vi "GA_Apply Elitism.vi"(6 "Parameters":T2={"Population size"=100, "Generations no."=500, "Significant digits"=4, "Crossover probabality"=0.85, "Mutation mode"=enum."one-point, fixed rate", "Use Gray code?"=FALSE, "Mutation rate"=0.05, "Min mutation rate"=0.0005, "Max mutation rate"=0.25, "Reproduction plan"=enum."Steady-state-replace-worst", "Elitism"=FALSE, "Fmax"=1} {"Max mutation rate" min=0.0 max=1.0; "Min mutation rate" min=0.0 max=1.0; "Mutation rate" min=0.0 max=1.0; "Crossover probabality" min=0.0 max=1.0; "Significant digits" min=1; "Generations no." min=1; "Population size" min=1}, 10 "Old Population":T1, 11 "Population in":T1) -> (3 "Population out":T1)   [LabVIEW 2016, in "Optimal Frequency Bands Search.lvlib" / "GeneticAlgorithm.lvlib"]
doc: "Применить элитизм. Оставить в популяции особей с лучшим значением функции приспособленности из предыдущего поколения"
uses:
  GeneticAlgorithm.lvlib
  GA_tParameters.ctl
  GA_tPopulation.ctl
panel:
  # "This VI is a part of BCI Design library, http://www.ru-bci.org \nCopyright © 2020, Sotnikov Peter, All rights reserved. License: GNU GPLv3"
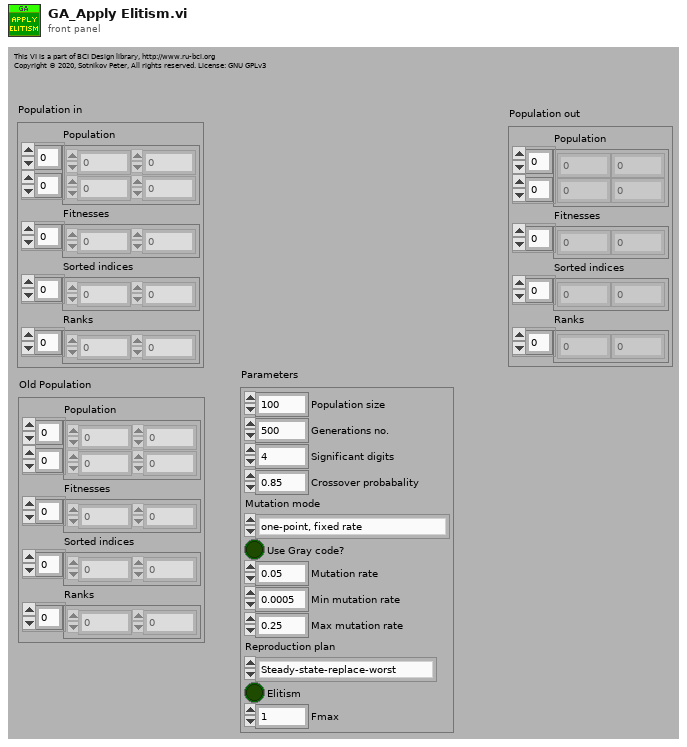
[diagram p1: front panel]
types:
  T1 = typedef "Optimal Frequency Bands Search.lvlib/GeneticAlgorithm.lvlib/GA_tPopulation.ctl" = cluster{"Population":i32[][], "Fitnesses":dbl[], "Sorted indices":i32[], "Ranks":i32[]}
  T2 = typedef "Optimal Frequency Bands Search.lvlib/GeneticAlgorithm.lvlib/GA_tParameters.ctl" = cluster{"Population size":i32, "Generations no.":i32, "Significant digits":i32, "Crossover probabality":dbl, "Mutation mode":enum16{"one-point, fixed rate", "one-point, fitness-adjustable rate", "one-point, distance-adjustable rate"}, "Use Gray code?":bool, "Mutation rate":dbl, "Min mutation rate":dbl, "Max mutation rate":dbl, "Reproduction plan":enum16{"Full generational replacement", "Steady-state-replace-random", "Steady-state-replace-worst"}, "Elitism":bool, "Fmax":i32}
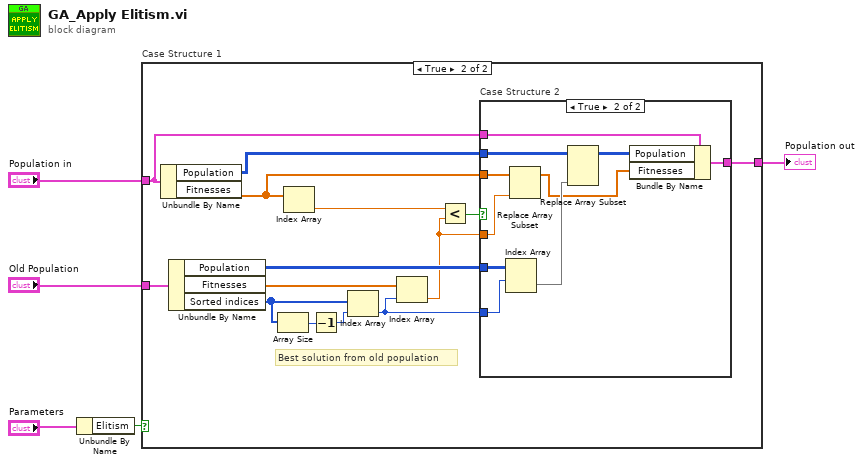
[diagram p0: block diagram]
diagram:
  n1 = Unbundle By Name("Parameters") -> ("Elitism"=w4:bool)
  n2 = case "Case Structure 1" shown="True" w4 {
    tunnel: "Population in" -> [w6 w14]
    tunnel: "Old Population" -> [_ w20]
    tunnel: [w6 w11] -> w1
    frame False {
    }
    frame True {
      # "Best solution from old population"
      n3 = Unbundle By Name(w14) -> ("Population"=w10:i32[][], "Fitnesses"=w7:dbl[])
      n4 = Unbundle By Name(w20) -> ("Population"=w13:i32[][], "Fitnesses"=w16:dbl[], "Sorted indices"=w19:i32[])
      n5 = Array Size(array=w19) -> (size(s)=w18:i32)
      n6 = Index Array(array=w7) -> (element=w9:dbl)  [unwired: 1 in]
      n7 = Decrement(x=w18) -> (x-1=w17:i32)
      n8 = Index Array(array=w19, index=w17) -> (element=w12:i32)
      n9 = Index Array(array=w16, index=w12) -> (element=w8:dbl)
      n10 = Less?(x=w9, y=w8) -> (x < y?=w15:bool)
      n11 = case "Case Structure 2" shown="True" w15 {
        tunnel: w10 -> [_ w29]
        tunnel: w14 -> [w21 w27]
        tunnel: w13 -> [_ w31]
        tunnel: w12 -> [_ w30]
        tunnel: [w21 w25] -> w11
        tunnel: w8 -> [_ w23]
        tunnel: w7 -> [_ w24]
        frame False {
        }
        frame True {
          n12 = Index Array "Index Array"(array=w31, index (row)=w30) -> (element=w28:i32[])  [unwired: 1 in]
          n13 = Replace Array Subset(array=w24, new element=w23) -> (w22:dbl[])  [unwired: 1 in]
          n14 = Replace Array Subset(array=w29, new element=w28) -> (w26:i32[][])  [unwired: 2 in]
          n15 = Bundle By Name(cluster=w27, "Population"=w26, "Fitnesses"=w22) -> (w25:T1)
        }
      }
    }
  }
  "Population out" <- w1
